vi "common_sensor_converter.vi"   [LabVIEW 2017, in "sensor_translation.lvlib"]
uses:
  sensor_translation.lvlib
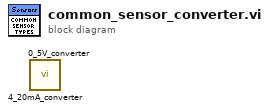
[diagram p0: block diagram]
diagram:
  n1 = call "4_20mA_converter.vi"() -> ()  [unwired: 3 in, 1 out]
  n2 = call "0_5V_converter.vi"() -> ()  [unwired: 3 in, 1 out]
